vi "一体站流程质控自动启动.vi"(6 "CODMn量程切换":enum32{"H", "L", "AUTO"}(ring)=enum."AUTO", 8 "总磷量程切换":enum32{"H", "L", "AUTO"}(ring)=enum."AUTO", 9 "总氮量程切换":enum32{"H", "L", "AUTO"}(ring)=enum."AUTO", 10 "氨氮量程切换":enum32{"H", "L", "AUTO"}(ring)=enum."AUTO", 11 "参数":T1={"是否启用仪器"=FALSE, "CODMn"={"启动测量模式"={"测量模式"=enum."水样测量"}, "确定按钮"=TRUE}, "启动模块"={"氨氮"=FALSE, "总磷"=FALSE, "总氮"=FALSE, "CODMn"=FALSE, "CODCr"=FALSE}, "常规启动"=FALSE, "直接启动"=FALSE}) -> ()   [LabVIEW 2016, in "质控单元.lvlib"]
uses:
  PLC/PLC.lvlib
panel:
  out "枚举 2":enum16{"初始化", "采配水启动", "等待", "配水", "排水", "结束"}(ring)
  out "枚举":enum16{"初始化", "采配水启动", "等待", "配水", "排水", "结束"}(ring)
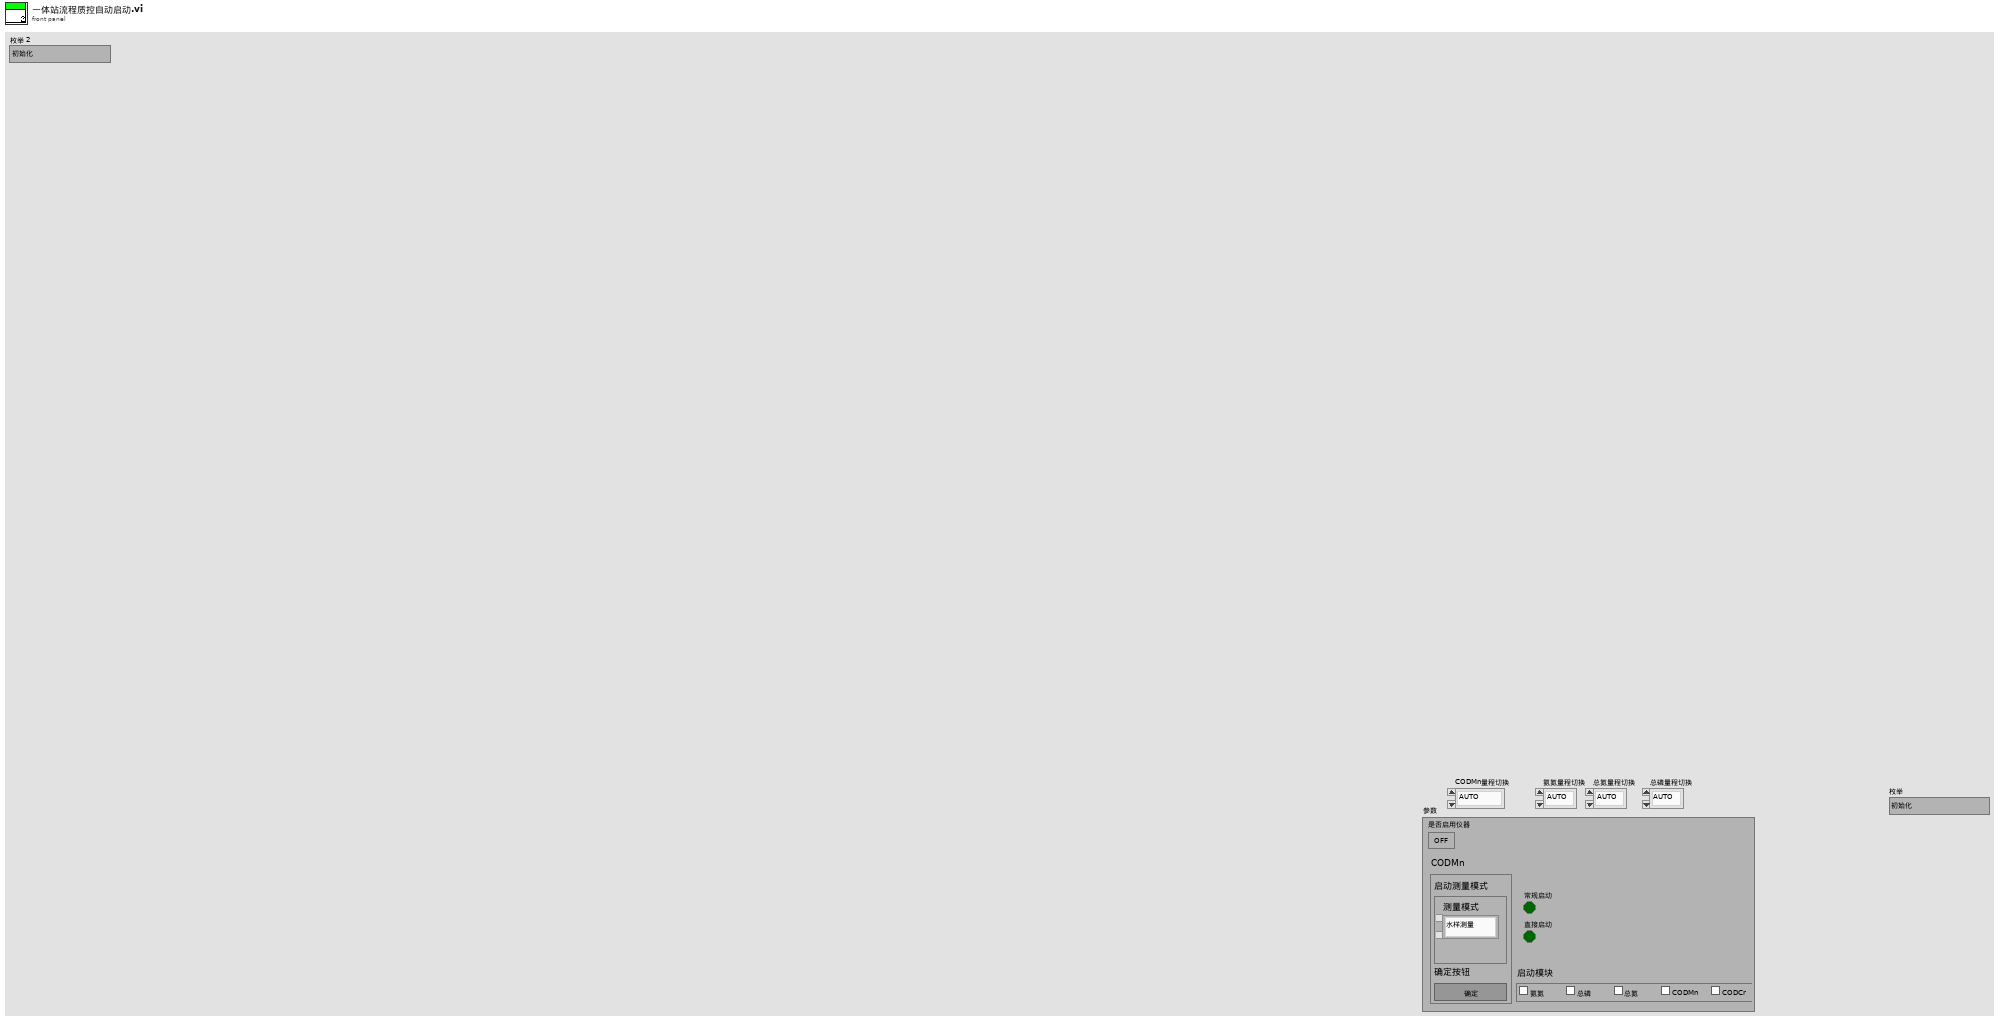
[diagram p1: front panel]
types:
  T1 = cluster{"是否启用仪器":bool, "CODMn":cluster{"启动测量模式":cluster{"测量模式":enum16{"水样测量", "标样核查", "加标回收", "平行样", "校零", "校标"}}, "确定按钮":bool}, "启动模块":cluster{"氨氮":bool, "总磷":bool, "总氮":bool, "CODMn":bool, "CODCr":bool}, "常规启动":bool, "直接启动":bool}
  T2 = cluster{"命令":string, cluster{"starting address":u16, "holding register value":u16}}
  T3 = cluster{"R0":i16, "R1":i16, "R2":i16, "R3":i16, "R4":i16, "R5":i16, "R6":i16, "R7":i16, "R8":i16, "R9":i16, "R10":i16, "R11":i16, "R12":i16, "R13":i16, "R14":i16, "R15":i16, "R16":i16, "R17":i16, "R18":i16, "R19":i16, "R20":i16, "R21":i16, "R22":i16, "R23":i16, "R24":i16, "R25":i16, "R26":i16, "R27":i16, "R28":i16, "R29":i16, "R30":i16, "R31":i16, "R32":i16, "R33":i16, "R34":i16, "R35":i16, "R36":i16, "R37":i16, "R38":i16, "R39":i16, "R40":i16, "R41":i16, "R42":i16, "R43":i16, "R44":i16, "R45":i16, "R46":i16, "R47":i16, "R48":i16, "R49":i16, "R50":i16, "R51":i16, "R52":i16, "R53":i16, "R54":i16, "R55":i16, "R56":i16}
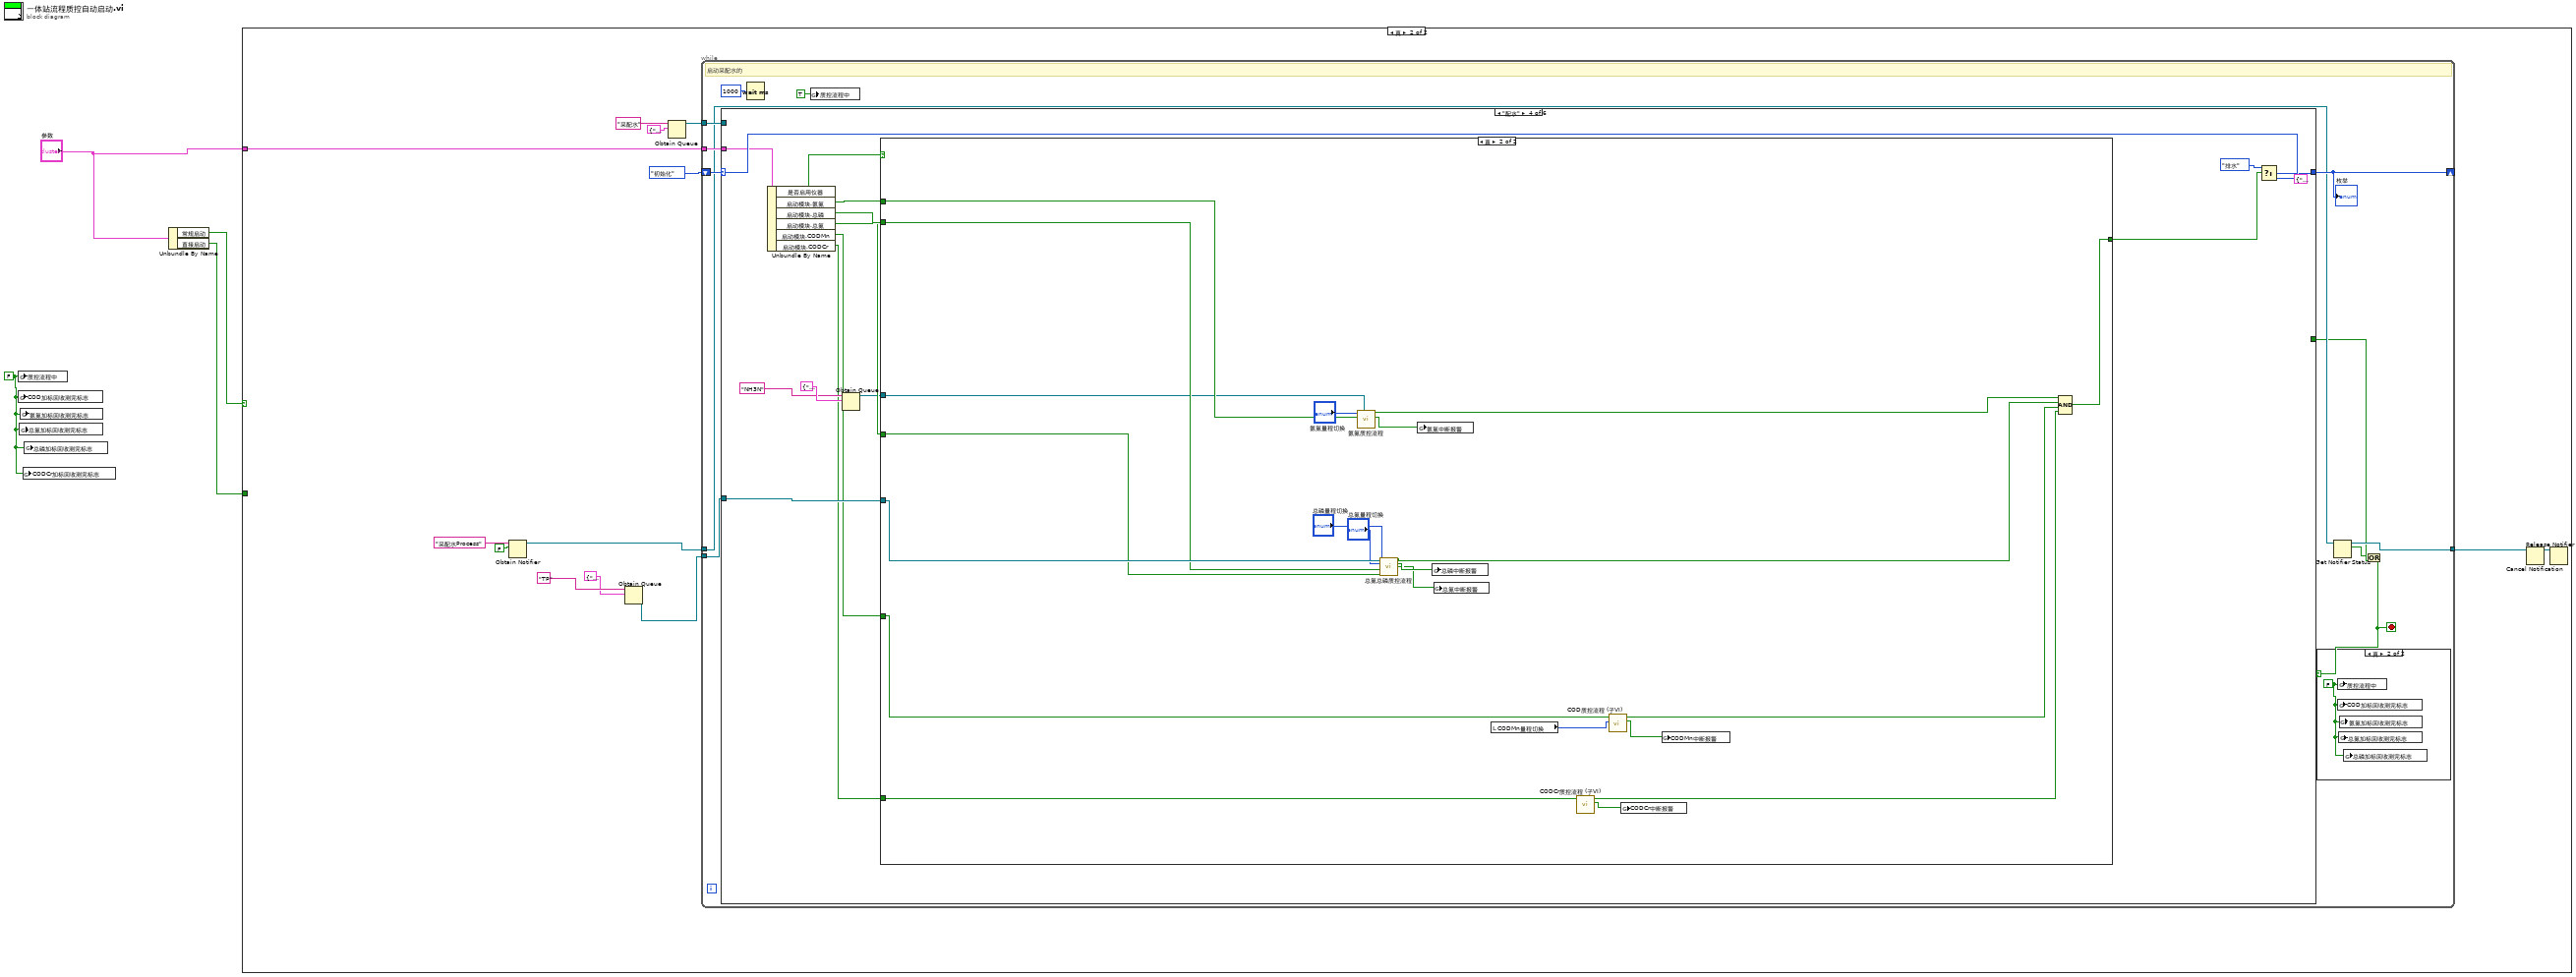
[diagram p0: block diagram]
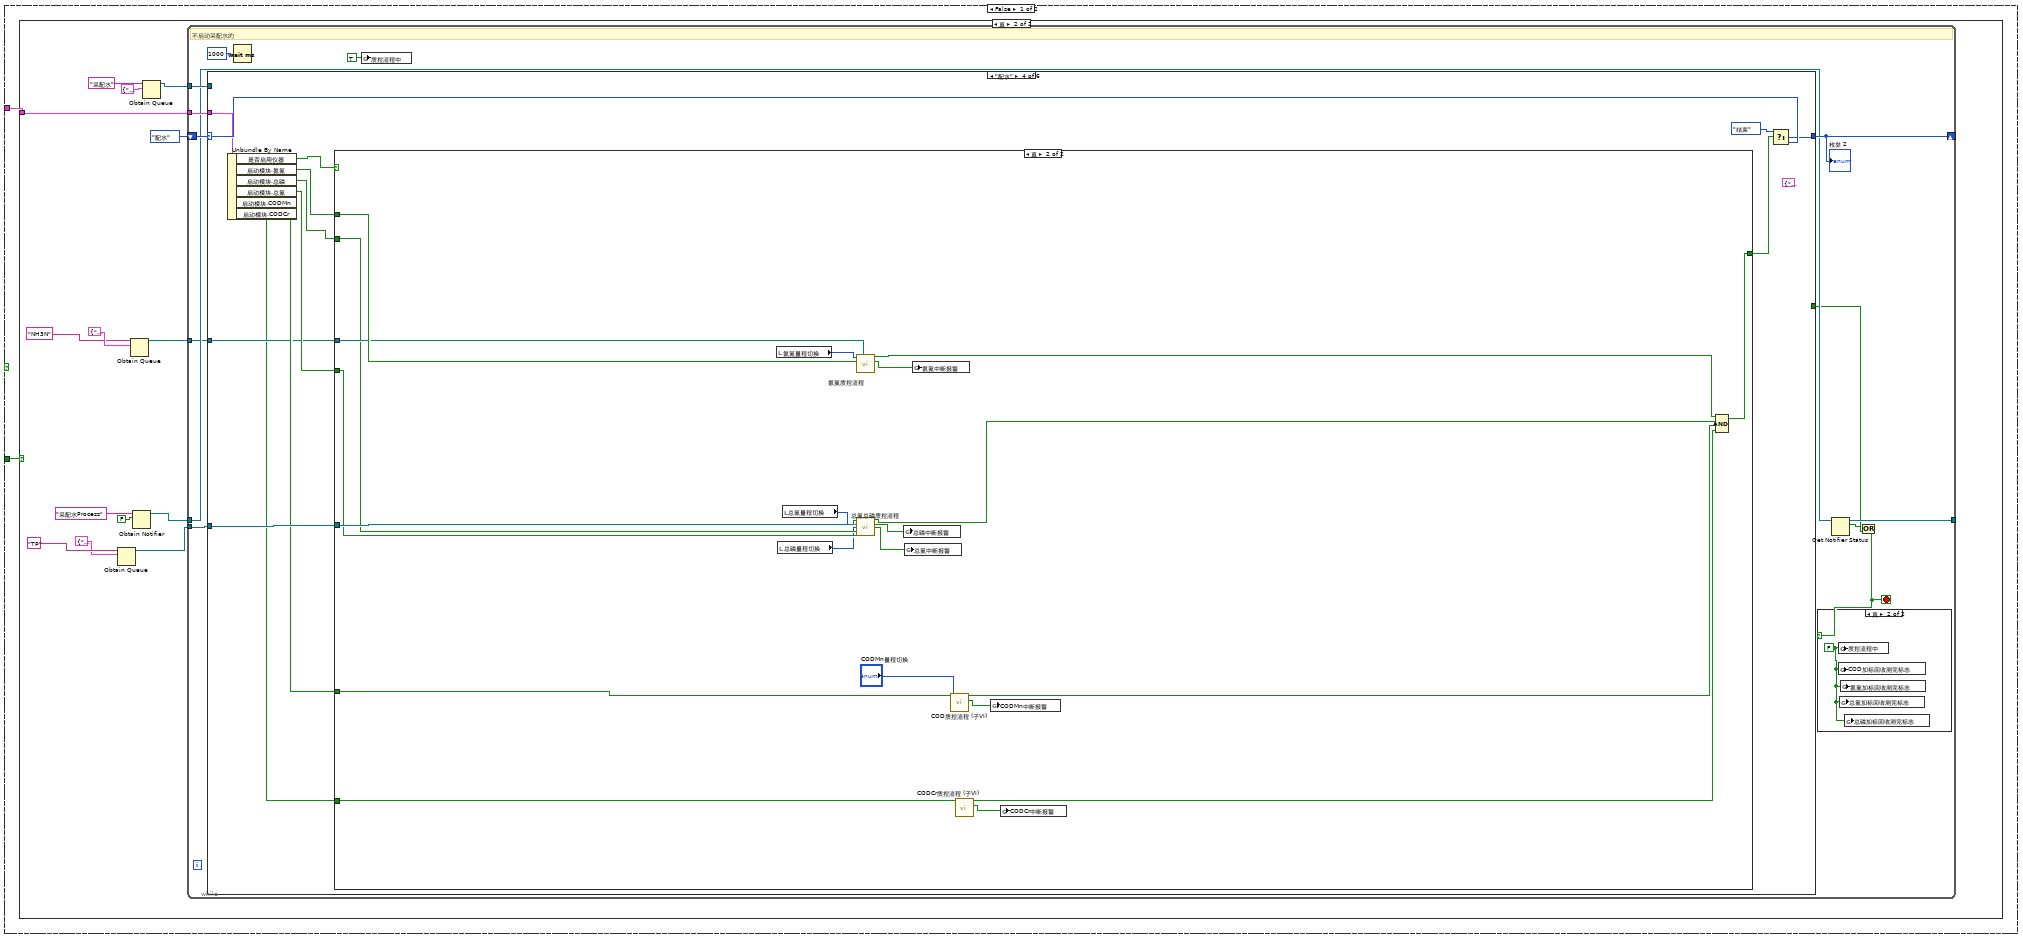
[diagram p2: hidden frame]
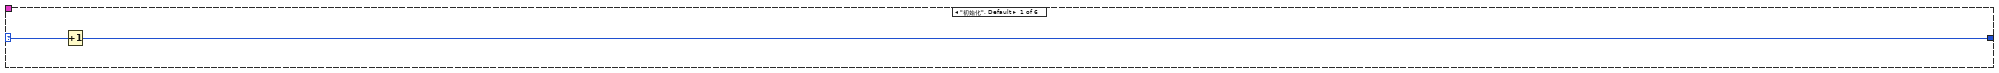
[diagram p5: hidden frame]
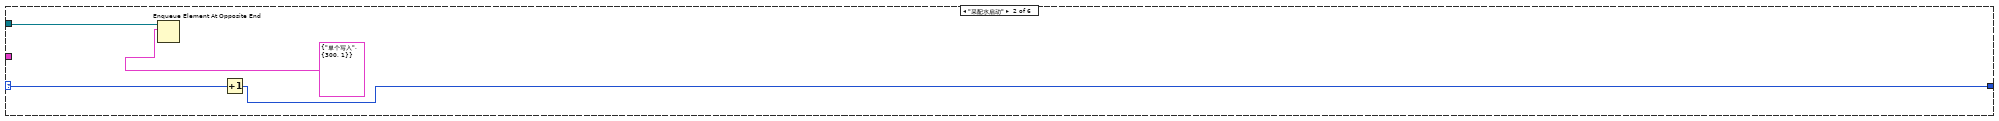
[diagram p6: hidden frame]
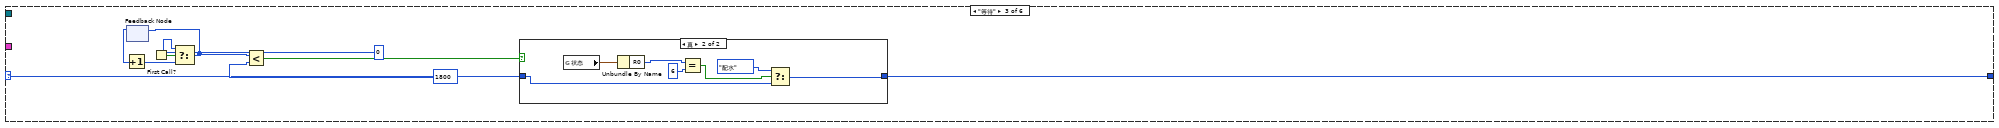
[diagram p7: hidden frame]
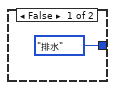
[diagram p8: hidden frame]
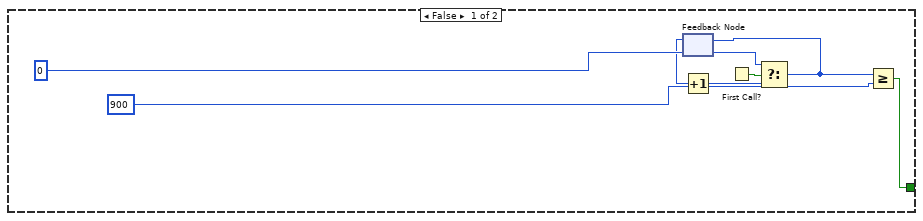
[diagram p9: hidden frame]
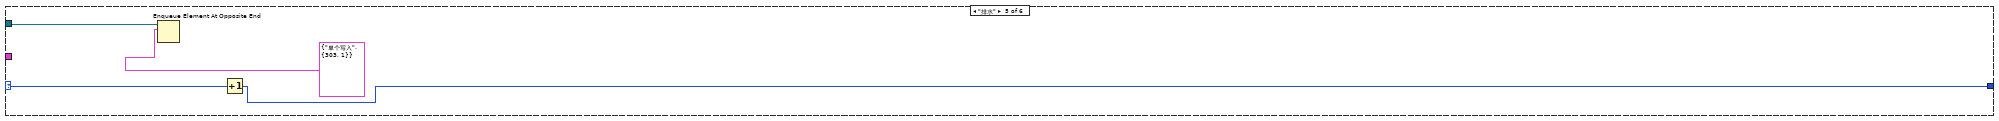
[diagram p10: hidden frame]
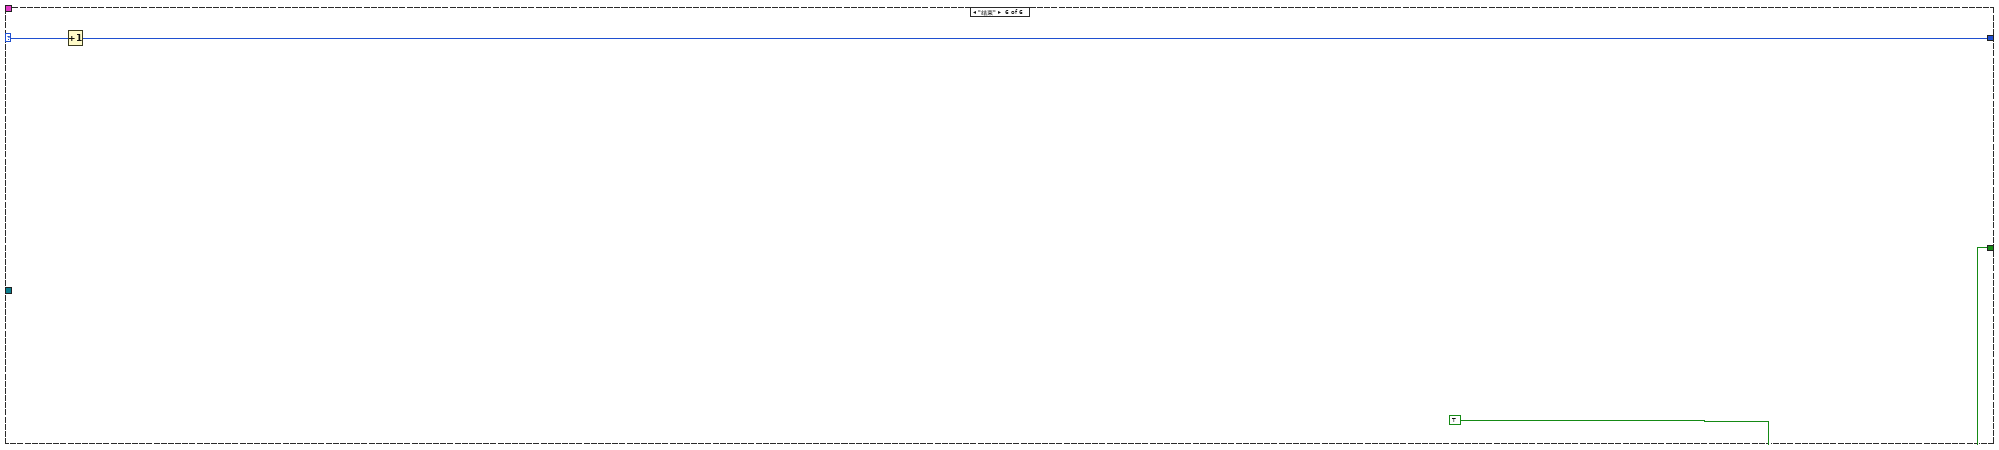
[diagram p11: hidden frame]
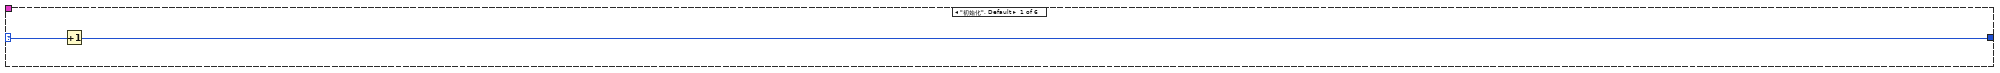
[diagram p13: hidden frame]
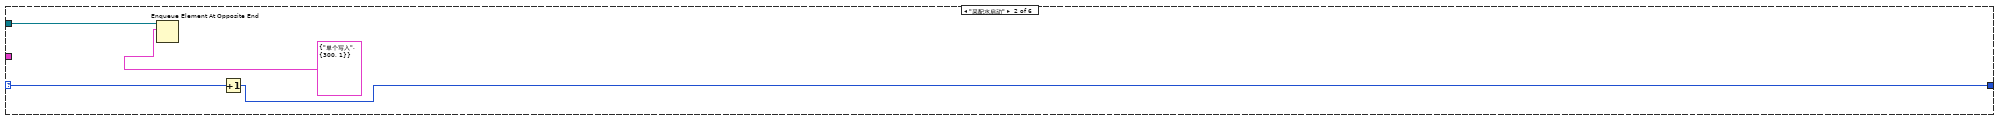
[diagram p14: hidden frame]
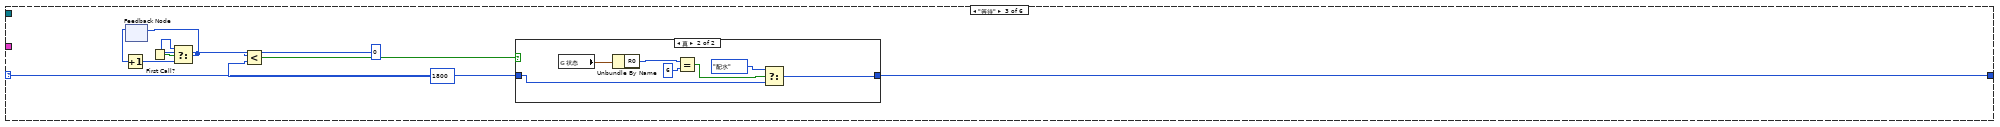
[diagram p15: hidden frame]
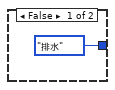
[diagram p16: hidden frame]
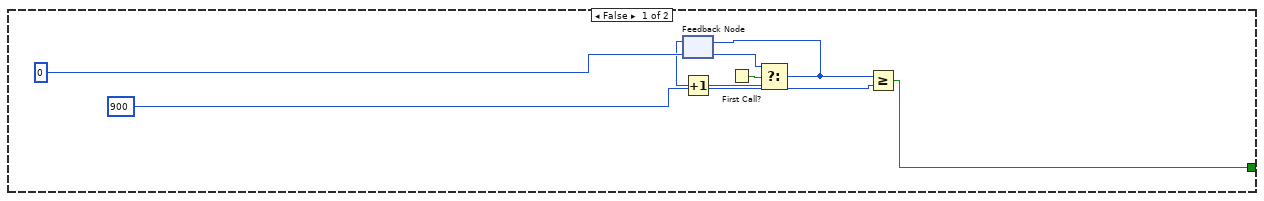
[diagram p17: hidden frame]
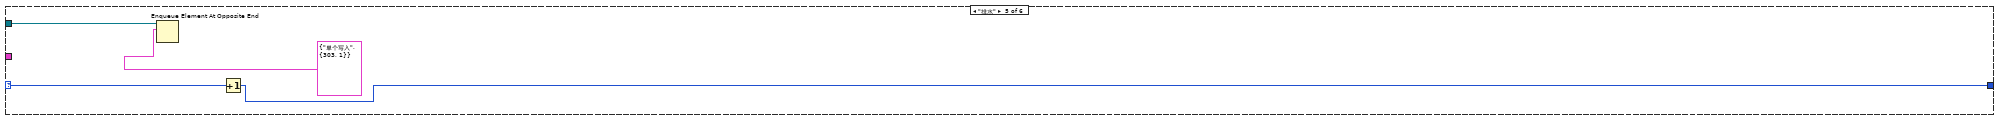
[diagram p18: hidden frame]
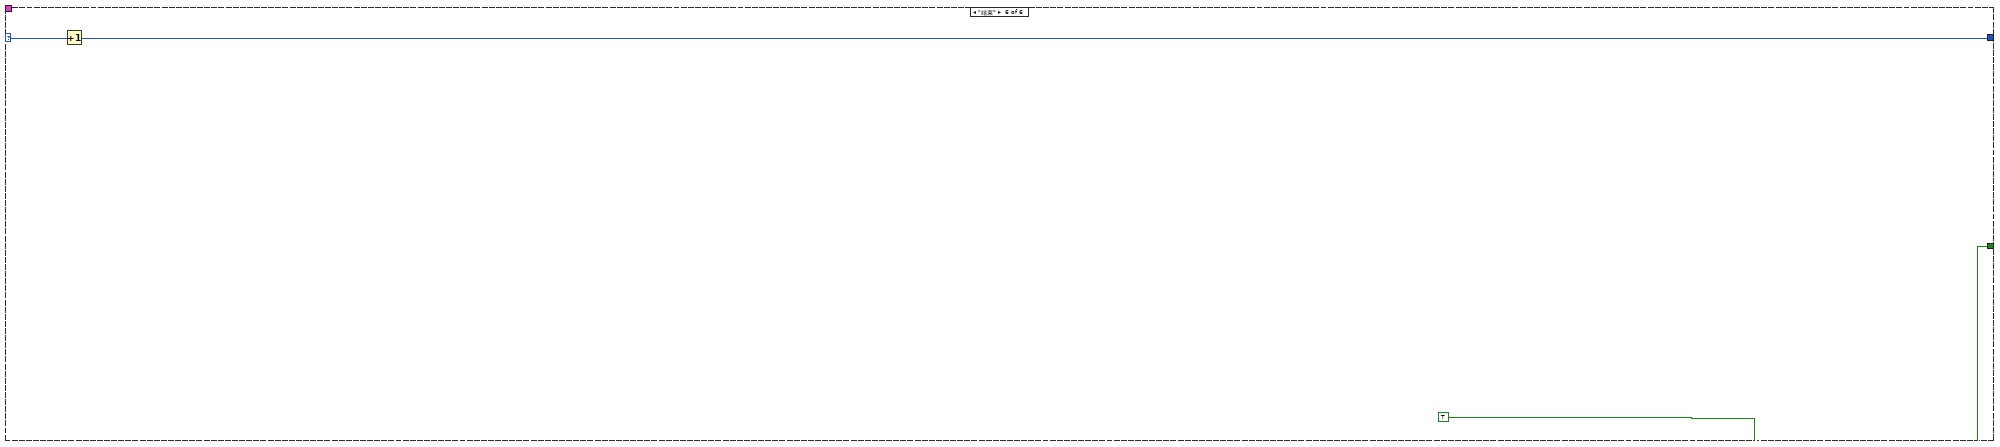
[diagram p19: hidden frame]
diagram:
  w1 = FALSE ("质控流程中")
  n1 = global write "质控测完标志全局 1.vi" "质控流程中"(w1) -> ()
  n2 = global write "质控测完标志全局 1.vi" "COD加标回收测完标志"(w1) -> ()
  n3 = global write "质控测完标志全局 1.vi" "总氮加标回收测完标志"(w1) -> ()
  n4 = global write "质控测完标志全局 1.vi" "氨氮加标回收测完标志"(w1) -> ()
  n5 = global write "质控测完标志全局 1.vi" "CODCr加标回收测完标志"(w1) -> ()
  n6 = global write "质控测完标志全局 1.vi" "总磷加标回收测完标志"(w1) -> ()
  n7 = Unbundle By Name("参数") -> ("常规启动"=w3:bool, "直接启动"=w2:bool)
  n8 = case shown="真" w3 {
    tunnel: "参数" -> [w5 w106]
    tunnel: w2 -> [w6 _]
    frame False {
      n9 = case shown="真" w6 {
        tunnel: w5 -> [_ w19]
        frame False {
        }
        frame True {
          n10 = Obtain Queue(name (unnamed)="TP" ("名称（未命名）"), element data type=cluster{"命令":string, "data":variant} {"命令"="", "data"=variant}) -> (queue out=w10:refnum<queue>)  [unwired: 3 in, 2 out]
          n11 = Obtain Queue(name (unnamed)="NH3N" ("名称（未命名）"), element data type=cluster{"命令":string, "data":variant} {"命令"="", "data"=variant}) -> (queue out=w7:refnum<queue>)  [unwired: 3 in, 2 out]
          n12 = Obtain Notifier(name (unnamed)="采配水Process" ("名称（未命名）"), notification data type=FALSE) -> (notifier out=w13:refnum<notifier>)  [unwired: 2 in, 2 out]
          n13 = Obtain Queue(name (unnamed)="采配水" ("名称（未命名）"), element data type=cluster{"命令":string, "数据":variant} {"命令"="", "数据"=variant}) -> (queue out=w16:refnum<queue>)  [unwired: 3 in, 2 out]
          n14 = while {
            tunnel: w16 -> [w33]
            shift-right: [w31] -> _
            shift-left: enum16{"初始化", "采配水启动", "等待", "配水", "排水", "结束"}."配水" ("枚举") -> [w32]
            tunnel: w10 -> [w29]
            tunnel: w19 -> [w28]
            tunnel: w13 -> [w27]
            tunnel: [w26] -> _
            tunnel: w7 -> [w23]
            stop <- w22 stop-if-true
            # "不启动采配水的"
            n15 = case shown="\"配水\"" w32 {
              selector: w32 -> [w36 w38 w47 w69 w100 w105]
              tunnel: w33 -> [_ w39 _ _ w101 _]
              tunnel: [w35 w37 w46 w68 w99 w104] -> w31
              tunnel: [_ _ _ _ _ TRUE] -> w25
              tunnel: w29 -> [_ _ _ w67 _ _]
              tunnel: w28 -> [_ _ _ w64 _ _]
              tunnel: w23 -> [_ _ _ w59 _ _]
              frame "初始化", Default {
                n16 = Increment(x=w36) -> (x+1=w35:enum16{"初始化", "采配水启动", "等待", "配水", "排水", "结束"})
              }
              frame "采配水启动" {
                n17 = Enqueue Element At Opposite End(queue=w39, element=T2 {"命令"="单个写入", {"starting address"=300, "holding register value"=1}} ("元素")) -> ()  [unwired: 2 in, 3 out]
                n18 = Increment(x=w38) -> (x+1=w37:enum16{"初始化", "采配水启动", "等待", "配水", "排水", "结束"})
              }
              frame "等待" {
                n19 = feedback #1() -> (w43:i32)  [unwired: 1 in]
                n20 = Increment(x=w43) -> (x+1=w42:i32)
                n21 = First Call?() -> (First Call?: T/F=w44:bool)
                n22 = Select(t=0, s=w44, f=w42) -> (s? t:f=w41:i32)
                n23 = feedback-in #1(w41) -> ()
                n24 = Less?(x=w41, y=1800) -> (x < y?=w48:bool)
                n25 = case shown="真" w48 {
                  tunnel: w47 -> [_ w52]
                  tunnel: [enum16{"初始化", "采配水启动", "等待", "配水", "排水", "结束"}."排水" ("枚举") w51] -> w46
                  frame False {
                  }
                  frame True {
                    n26 = global read "采配水全局变量.vi" "状态"() -> (w57:T3)
                    n27 = Unbundle By Name(w57) -> ("R0"=w56:i16)
                    n28 = Equal?(x=w56, y=i16 6) -> (x = y?=w54:bool)
                    n29 = Select(t=enum16{"初始化", "采配水启动", "等待", "配水", "排水", "结束"}."配水" ("枚举"), s=w54, f=w52) -> (s? t:f=w51:enum16{"初始化", "采配水启动", "等待", "配水", "排水", "结束"})
                  }
                }
              }
              frame "配水" {
                (unwired) cluster{"命令":string, "data":variant} {"命令"="启动", "data"=variant(cluster{"站号":u16, "控制命令输出":u16[]} {"站号"=1, "控制命令输出"=[256, 0]})} ("元素")
                n30 = Unbundle By Name(w64) -> ("是否启用仪器"=w66:bool, "启动模块.氨氮"=w62:bool, "启动模块.总磷"=w63:bool, "启动模块.总氮"=w60:bool, "启动模块.CODMn"=w61:bool, "启动模块.CODCr"=w58:bool)
                n31 = case shown="真" w66 {
                  tunnel: w67 -> [_ w92]
                  tunnel: [w71 w98] -> w65
                  tunnel: w63 -> [_ w91]
                  tunnel: w62 -> [_ w97]
                  tunnel: w61 -> [_ w96]
                  tunnel: w60 -> [_ w90]
                  tunnel: w59 -> [_ w94]
                  tunnel: w58 -> [_ w80]
                  frame False {
                    n32 = feedback #2() -> (w75:i32)  [unwired: 1 in]
                    n33 = Increment(x=w75) -> (x+1=w74:i32)
                    n34 = First Call?() -> (First Call?: T/F=w76:bool)
                    n35 = Select(t=0, s=w76, f=w74) -> (s? t:f=w72:i32)
                    n36 = feedback-in #2(w72) -> ()
                    n37 = Greater Or Equal?(x=w72, y=900) -> (x >= y?=w71:bool)
                  }
                  frame True {
                    n38 = local read "氨氮量程切换"() -> (w84:enum32{"H", "L", "AUTO"})
                    n39 = local read "总磷量程切换"() -> (w86:enum32{"H", "L", "AUTO"})
                    n40 = local read "总氮量程切换"() -> (w85:enum32{"H", "L", "AUTO"})
                    n41 = call "氨氮质控流程.vi"("队列输入NH3"=w94, "氨氮"=w97, "氨氮量程切换"=w84) -> ("氨氮中断报警"=w83:bool, "布尔"=w95:bool)  [unwired: 7 in]
                    n42 = call "总氮总磷质控流程.vi"("队列输入TP"=w92, "总氮量程切换"=w85, "总磷量程切换"=w86, "总磷"=w91, "总氮"=w90) -> ("布尔"=w89:bool, "总磷中断报警"=w82:bool, "总氮中断报警"=w81:bool)  [unwired: 8 in]
                    n43 = global write "质控中断报警全局.vi" "总磷中断报警"(w82) -> ()
                    n44 = global write "质控中断报警全局.vi" "总氮中断报警"(w81) -> ()
                    n45 = global write "质控中断报警全局.vi" "氨氮中断报警"(w83) -> ()
                    n46 = call "COD质控流程 (子VI).vi"("CODMn量程切换"="CODMn量程切换", "COD"=w96) -> ("CODMn中断报警"=w87:bool, "布尔"=w93:bool)  [unwired: 8 in]
                    n47 = call "CODCr质控流程 (子VI).vi"("CODCr"=w80) -> ("CODCr中断报警"=w79:bool, "布尔"=w78:bool)  [unwired: 9 in]
                    n48 = global write "质控中断报警全局.vi" "CODMn中断报警"(w87) -> ()
                    n49 = global write "质控中断报警全局.vi" "CODCr中断报警"(w79) -> ()
                    n50 = Compound Arithmetic op=AND ("复合运算")(w95, w89, w93, w78) -> (w98:bool)
                  }
                }
                n51 = Select(t=enum16{"初始化", "采配水启动", "等待", "配水", "排水", "结束"}."结束" ("枚举"), s=w65, f=w69) -> (s? t:f=w68:enum16{"初始化", "采配水启动", "等待", "配水", "排水", "结束"})
              }
              frame "排水" {
                n52 = Enqueue Element At Opposite End(queue=w101, element=T2 {"命令"="单个写入", {"starting address"=303, "holding register value"=1}} ("元素")) -> ()  [unwired: 2 in, 3 out]
                n53 = Increment(x=w100) -> (x+1=w99:enum16{"初始化", "采配水启动", "等待", "配水", "排水", "结束"})
              }
              frame "结束" {
                n54 = Increment(x=w105) -> (x+1=w104:enum16{"初始化", "采配水启动", "等待", "配水", "排水", "结束"})
              }
            }
            "枚举 2" <- w31
            n55 = Wait (ms)(milliseconds to wait=u32 1000 ("等待时间（毫秒）")) -> ()  [unwired: 1 out]
            n56 = global write "质控测完标志全局 1.vi" "质控流程中"(TRUE ("质控流程中")) -> ()
            n57 = Get Notifier Status(notifier=w27) -> (notifier out=w26:refnum<notifier>, current notification=w24:bool)  [unwired: 1 in, 3 out]
            n58 = Or(x=w24, y=w25) -> (x .or. y?=w22:bool)
            n59 = case shown="真" w22 {
              frame False {
              }
              frame True {
                w34 = FALSE ("质控流程中")
                n60 = global write "质控测完标志全局 1.vi" "质控流程中"(w34) -> ()
                n61 = global write "质控测完标志全局 1.vi" "COD加标回收测完标志"(w34) -> ()
                n62 = global write "质控测完标志全局 1.vi" "总氮加标回收测完标志"(w34) -> ()
                n63 = global write "质控测完标志全局 1.vi" "氨氮加标回收测完标志"(w34) -> ()
                n64 = global write "质控测完标志全局 1.vi" "总磷加标回收测完标志"(w34) -> ()
              }
            }
          }
        }
      }
    }
    frame True {
      n65 = Obtain Notifier(name (unnamed)="采配水Process" ("名称（未命名）"), notification data type=FALSE) -> (notifier out=w109:refnum<notifier>)  [unwired: 2 in, 2 out]
      n66 = Obtain Queue(name (unnamed)="TP" ("名称（未命名）"), element data type=cluster{"命令":string, "data":variant} {"命令"="", "data"=variant}) -> (queue out=w112:refnum<queue>)  [unwired: 3 in, 2 out]
      n67 = Obtain Queue(name (unnamed)="采配水" ("名称（未命名）"), element data type=cluster{"命令":string, "数据":variant} {"命令"="", "数据"=variant}) -> (queue out=w116:refnum<queue>)  [unwired: 3 in, 2 out]
      n68 = while {
        tunnel: w116 -> [w130]
        shift-right: [w128] -> _
        shift-left: enum16{"初始化", "采配水启动", "等待", "配水", "排水", "结束"}."初始化" ("枚举") -> [w129]
        tunnel: w112 -> [w126]
        tunnel: w106 -> [w125]
        tunnel: w109 -> [w124]
        tunnel: [w123] -> w108
        stop <- w120 stop-if-true
        # "启动采配水的"
        n69 = case shown="\"配水\"" w129 {
          selector: w129 -> [w133 w135 w144 w168 w199 w204]
          tunnel: w130 -> [_ w136 _ _ w200 _]
          tunnel: [w132 w134 w143 w167 w198 w203] -> w128
          tunnel: [_ _ _ _ _ TRUE] -> w122
          tunnel: w126 -> [_ _ _ w166 _ _]
          tunnel: w125 -> [_ _ _ w163 _ _]
          frame "初始化", Default {
            n70 = Increment(x=w133) -> (x+1=w132:enum16{"初始化", "采配水启动", "等待", "配水", "排水", "结束"})
          }
          frame "采配水启动" {
            n71 = Enqueue Element At Opposite End(queue=w136, element=T2 {"命令"="单个写入", {"starting address"=300, "holding register value"=1}} ("元素")) -> ()  [unwired: 2 in, 3 out]
            n72 = Increment(x=w135) -> (x+1=w134:enum16{"初始化", "采配水启动", "等待", "配水", "排水", "结束"})
          }
          frame "等待" {
            n73 = feedback #3() -> (w140:i32)  [unwired: 1 in]
            n74 = Increment(x=w140) -> (x+1=w139:i32)
            n75 = First Call?() -> (First Call?: T/F=w141:bool)
            n76 = Select(t=0, s=w141, f=w139) -> (s? t:f=w138:i32)
            n77 = feedback-in #3(w138) -> ()
            n78 = Less?(x=w138, y=1800) -> (x < y?=w145:bool)
            n79 = case shown="真" w145 {
              tunnel: w144 -> [_ w149]
              tunnel: [enum16{"初始化", "采配水启动", "等待", "配水", "排水", "结束"}."排水" ("枚举") w148] -> w143
              frame False {
              }
              frame True {
                n80 = global read "采配水全局变量.vi" "状态"() -> (w154:T3)
                n81 = Unbundle By Name(w154) -> ("R0"=w153:i16)
                n82 = Equal?(x=w153, y=i16 6) -> (x = y?=w151:bool)
                n83 = Select(t=enum16{"初始化", "采配水启动", "等待", "配水", "排水", "结束"}."配水" ("枚举"), s=w151, f=w149) -> (s? t:f=w148:enum16{"初始化", "采配水启动", "等待", "配水", "排水", "结束"})
              }
            }
          }
          frame "配水" {
            (unwired) cluster{"命令":string, "data":variant} {"命令"="启动", "data"=variant(cluster{"站号":u16, "控制命令输出":u16[]} {"站号"=1, "控制命令输出"=[256, 0]})} ("元素")
            n84 = Unbundle By Name(w163) -> ("是否启用仪器"=w165:bool, "启动模块.氨氮"=w161:bool, "启动模块.总磷"=w162:bool, "启动模块.总氮"=w159:bool, "启动模块.CODMn"=w160:bool, "启动模块.CODCr"=w155:bool)
            n85 = Obtain Queue(name (unnamed)="NH3N" ("名称（未命名）"), element data type=cluster{"命令":string, "data":variant} {"命令"="", "data"=variant}) -> (queue out=w156:refnum<queue>)  [unwired: 3 in, 2 out]
            n86 = case shown="真" w165 {
              tunnel: w166 -> [_ w192]
              tunnel: [w170 w196] -> w164
              tunnel: w162 -> [_ w191]
              tunnel: w161 -> [_ w195]
              tunnel: w160 -> [_ w194]
              tunnel: w159 -> [_ w190]
              tunnel: w156 -> [_ w188]
              tunnel: w155 -> [_ w178]
              frame False {
                n87 = feedback #4() -> (w174:i32)  [unwired: 1 in]
                n88 = Increment(x=w174) -> (x+1=w173:i32)
                n89 = First Call?() -> (First Call?: T/F=w175:bool)
                n90 = Select(t=0, s=w175, f=w173) -> (s? t:f=w171:i32)
                n91 = feedback-in #4(w171) -> ()
                n92 = Greater Or Equal?(x=w171, y=900) -> (x >= y?=w170:bool)
              }
              frame True {
                n93 = call "氨氮质控流程.vi"("队列输入NH3"=w188, "氨氮"=w195, "氨氮量程切换"="氨氮量程切换") -> ("氨氮中断报警"=w180:bool, "布尔"=w197:bool)  [unwired: 7 in]
                n94 = call "总氮总磷质控流程.vi"("队列输入TP"=w192, "总氮量程切换"="总氮量程切换", "总磷量程切换"="总磷量程切换", "总磷"=w191, "总氮"=w190) -> ("布尔"=w189:bool, "总磷中断报警"=w182:bool, "总氮中断报警"=w181:bool)  [unwired: 8 in]
                n95 = global write "质控中断报警全局.vi" "氨氮中断报警"(w180) -> ()
                n96 = global write "质控中断报警全局.vi" "总磷中断报警"(w182) -> ()
                n97 = global write "质控中断报警全局.vi" "总氮中断报警"(w181) -> ()
                n98 = local read "CODMn量程切换"() -> (w187:enum32{"H", "L", "AUTO"})
                n99 = call "CODCr质控流程 (子VI).vi"("CODCr"=w178) -> ("CODCr中断报警"=w179:bool, "布尔"=w177:bool)  [unwired: 9 in]
                n100 = call "COD质控流程 (子VI).vi"("CODMn量程切换"=w187, "COD"=w194) -> ("CODMn中断报警"=w186:bool, "布尔"=w193:bool)  [unwired: 8 in]
                n101 = global write "质控中断报警全局.vi" "CODCr中断报警"(w179) -> ()
                n102 = global write "质控中断报警全局.vi" "CODMn中断报警"(w186) -> ()
                n103 = Compound Arithmetic op=AND ("复合运算")(w197, w189, w193, w177) -> (w196:bool)
              }
            }
            n104 = Select(t=enum16{"初始化", "采配水启动", "等待", "配水", "排水", "结束"}."排水" ("枚举"), s=w164, f=w168) -> (s? t:f=w167:enum16{"初始化", "采配水启动", "等待", "配水", "排水", "结束"})
          }
          frame "排水" {
            n105 = Enqueue Element At Opposite End(queue=w200, element=T2 {"命令"="单个写入", {"starting address"=303, "holding register value"=1}} ("元素")) -> ()  [unwired: 2 in, 3 out]
            n106 = Increment(x=w199) -> (x+1=w198:enum16{"初始化", "采配水启动", "等待", "配水", "排水", "结束"})
          }
          frame "结束" {
            n107 = Increment(x=w204) -> (x+1=w203:enum16{"初始化", "采配水启动", "等待", "配水", "排水", "结束"})
          }
        }
        "枚举" <- w128
        n108 = Wait (ms)(milliseconds to wait=u32 1000 ("等待时间（毫秒）")) -> ()  [unwired: 1 out]
        n109 = global write "质控测完标志全局 1.vi" "质控流程中"(TRUE ("质控流程中")) -> ()
        n110 = Get Notifier Status(notifier=w124) -> (notifier out=w123:refnum<notifier>, current notification=w121:bool)  [unwired: 1 in, 3 out]
        n111 = Or(x=w121, y=w122) -> (x .or. y?=w120:bool)
        n112 = case shown="真" w120 {
          frame False {
          }
          frame True {
            w131 = FALSE ("质控流程中")
            n113 = global write "质控测完标志全局 1.vi" "质控流程中"(w131) -> ()
            n114 = global write "质控测完标志全局 1.vi" "COD加标回收测完标志"(w131) -> ()
            n115 = global write "质控测完标志全局 1.vi" "总氮加标回收测完标志"(w131) -> ()
            n116 = global write "质控测完标志全局 1.vi" "氨氮加标回收测完标志"(w131) -> ()
            n117 = global write "质控测完标志全局 1.vi" "总磷加标回收测完标志"(w131) -> ()
          }
        }
      }
      n118 = Cancel Notification(0:w108) -> (8:w107:refnum<notifier>)  [unwired: 1 in, 2 out]
      n119 = Release Notifier(notifier=w107) -> ()  [unwired: 2 in, 3 out]
    }
  }
